vi "iniSubsciberDevice.vi"(6 "DeviceName":string, 8 "error in (no error)":errorcluster, 11 "variant":variant) -> (0 "error out":errorcluster, 3 "Subscriber cluster":T1)   [LabVIEW 2011]
uses:
  SubscriberCluster_TypDEf.ctl
  tcp_new_data_event.ctl
  tcp new data cluster.ctl
panel:
  out "all lower case string":string[](array[string])
  out "Devices":string[](array[string])
  out "Element Names":string[](array[string])
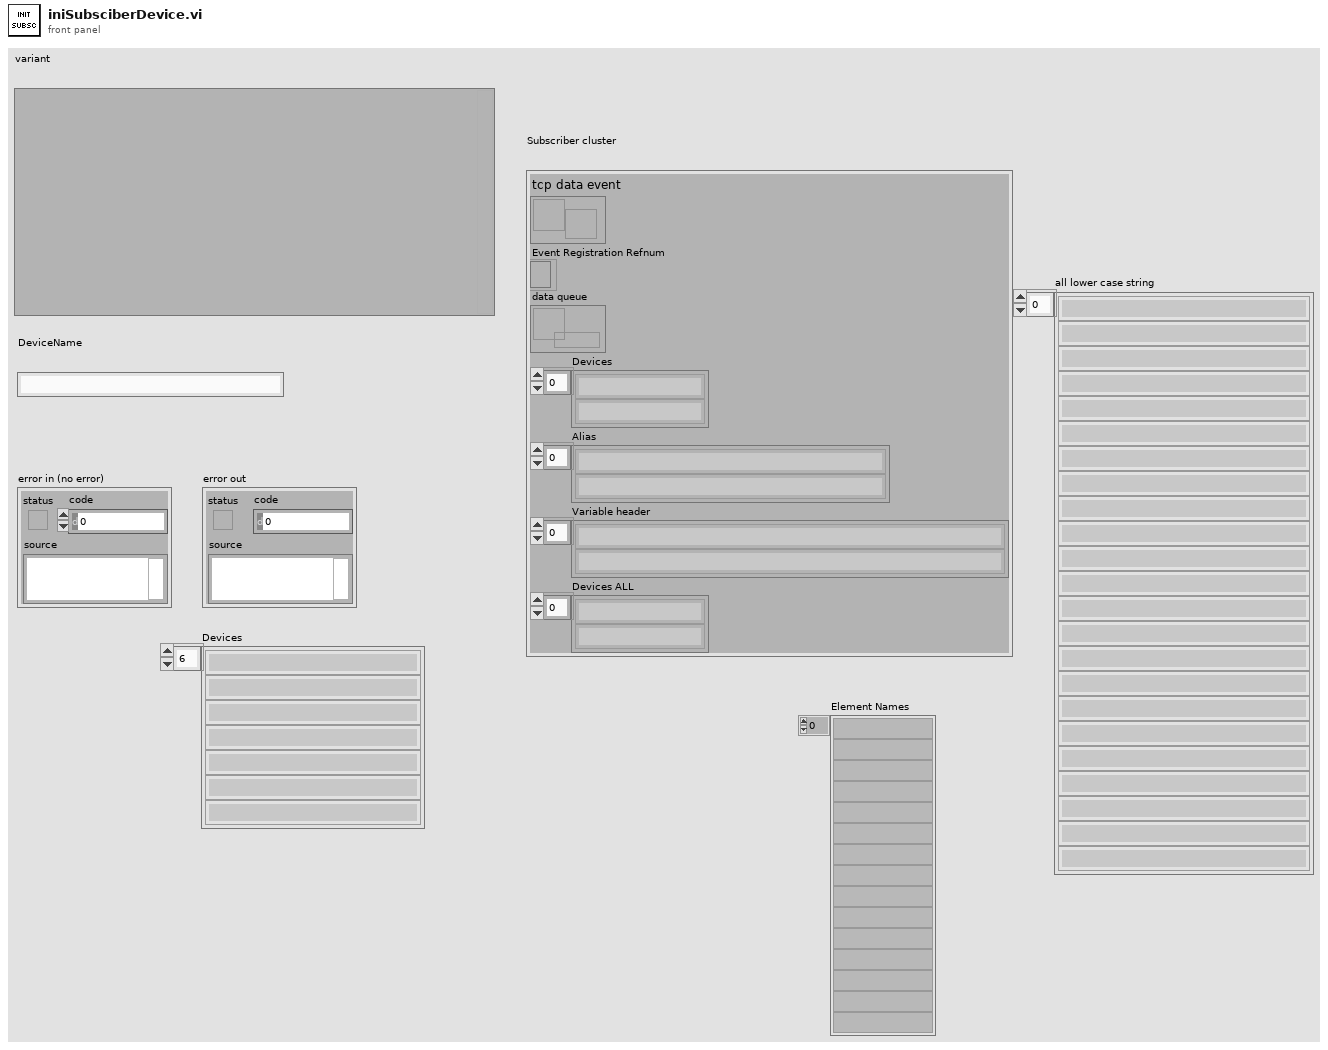
[diagram p1: front panel]
types:
  T1 = typedef "SubscriberCluster_TypDEf.ctl" = cluster{"tcp data event":T2, "Event Registration Refnum":refnum<event-registration>, "data queue":refnum<queue>, "Devices":string[], "Alias":string[], "Variable header":string[], "Devices ALL":string[]}
  T2 = typedef "tcp_new_data_event.ctl" = refnum<user-event>
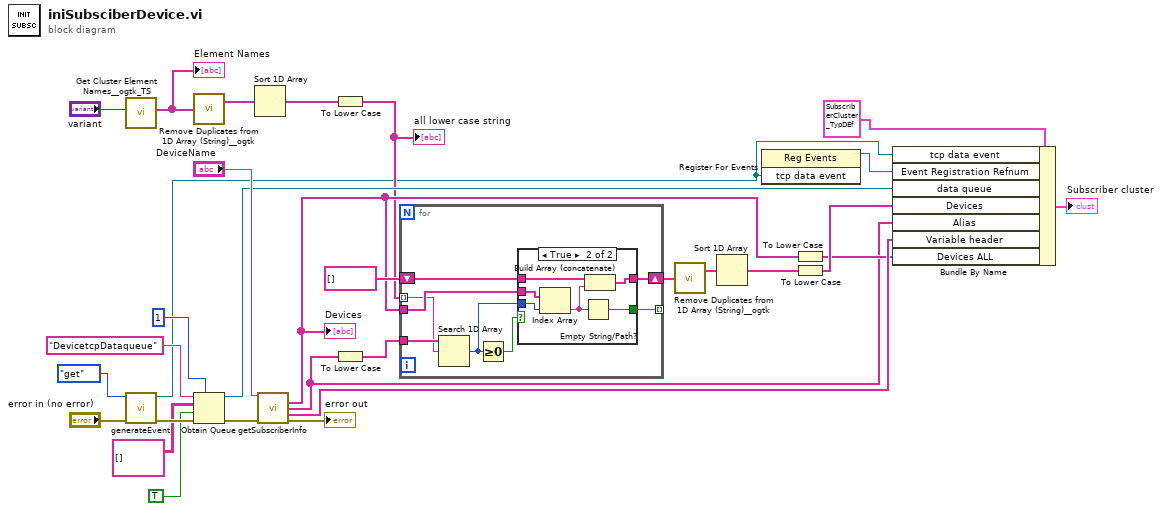
[diagram p0: block diagram]
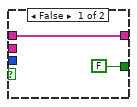
[diagram p2: hidden frame]
diagram:
  n1 = call "Get Cluster Element Names__ogtk_TS.vi"("Variant"="variant") -> ("Names (Array)"=w2:string[])  [unwired: 9 in, 1 out]
  "Element Names" <- w2
  n2 = call "generateEvent.vi"("error in"="error in (no error)", "command"=enum16{"ini", "get", "close"}."get") -> ("error out"=w22:errorcluster, "tcp data event"=w1:T2)  [unwired: 8 in]
  n3 = call "Remove Duplicates from 1D Array (String)__ogtk.vi"("Input Array"=w2) -> ("Output Array"=w14:string[])  [unwired: 1 out]
  n4 = Obtain Queue(max queue size (-1, unlimited)=1, name (unnamed)="DevicetcpDataqueue", element data type=string[][] [] ("Data in"), create if not found? (T)=TRUE, error in (no error)=w22) -> (queue out=w23:refnum<queue>, error out=w26:errorcluster)  [unwired: 1 out]
  n5 = Sort 1D Array(array=w14) -> (sorted array=w5:string[])
  n6 = call "getSubscriberInfo.vi"("DeviceName"="DeviceName", "error in (no error)"=w26) -> ("Devices"=w8:string[], "Alias"=w6:string[], "Variable header"=w25:string[], "error out"=→"error out":errorcluster)  [unwired: 9 in, 1 out]
  "Devices" <- w8
  n7 = To Lower Case(string=w5) -> (all lower case string=w4:string[])
  "all lower case string" <- w4
  n8 = To Lower Case(string=w6) -> (all lower case string=w9:string[])
  n9 = for {
    tunnel: w4 -> [w31] mode=indexing
    tunnel: w9 -> [w38]
    tunnel: w8 -> [w37]
    shift-right: [w34] -> w12
    shift-left: string[] [] -> [w33]
    tunnel: [w32] -> _ mode=indexing
    n10 = Search 1D Array(1D array=w38, element=w31) -> (index of element=w35:i32)  [unwired: 1 in]
    n11 = Greater Or Equal To 0?(x=w35) -> (x >= 0?=w36:bool)
    n12 = case shown="True" w36 {
      tunnel: w37 -> [_ w46]
      tunnel: w35 -> [_ w45]
      tunnel: [w40 w44] -> w34
      tunnel: w33 -> [w40 w43]
      tunnel: [FALSE w41] -> w32
      frame False {
      }
      frame True {
        n13 = Index Array(array=w46, index=w45) -> (element=w42:string)
        n14 = Empty String/Path?(string/path=w42) -> (empty?=w41:bool)
        n15 = Build Array (concatenate)(w43, w42) -> (w44:string[])
      }
    }
  }
  n16 = call "Remove Duplicates from 1D Array (String)__ogtk.vi"("Input Array"=w12) -> ("Output Array"=w11:string[])  [unwired: 1 out]
  n17 = Sort 1D Array(array=w11) -> (sorted array=w10:string[])
  n18 = register-events(w1) -> (reference out=w17:refnum<event-registration>)  [unwired: 2 in, 1 out]
  n19 = To Lower Case(string=w8) -> (all lower case string=w7:string[])
  n20 = To Lower Case(string=w10) -> (all lower case string=w28:string[])
  n21 = Bundle By Name(cluster=T1 {"tcp data event"=refnum, "Event Registration Refnum"=refnum, "data queue"=refnum, "Devices"=[], "Alias"=[], "Variable header"=[], "Devices ALL"=[]} ("SubscriberCluster"), "tcp data event"=w1, "Event Registration Refnum"=w17, "data queue"=w23, "Devices"=w28, "Alias"=w6, "Variable header"=w25, "Devices ALL"=w7) -> (→"Subscriber cluster":T1)
